vi "VCI_UsbDeviceReset.vi"(8 "error in (no error)":errorcluster caption="错误输入（无错误）", 9 "Reserved":u32, 10 "DevIndex":u32, 11 "DevType":T1=2 items=["USB-CAN"=2, "USB-CAN2"=3]) -> (0 "error out":errorcluster caption="错误输出", 3 "Return Val":T2=1 items=["OK"=1, "ERROR1"=0, "ERROR2"=-1])   [LabVIEW 2018, in "ControlCan.lvlib"]
uses:
  ControlCan.lvlib
  Return Val.ctl
  DevType.ctl
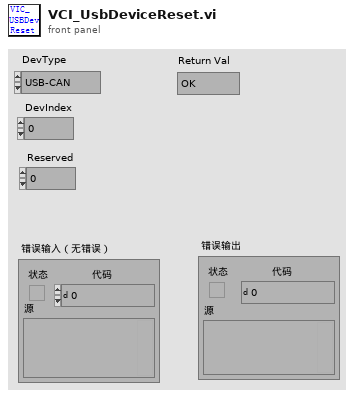
[diagram p1: front panel]
types:
  T1 = typedef "ControlCAN.lvlib/DevType.ctl" = u32
  T2 = typedef "ControlCAN.lvlib/Return Val.ctl" = i32
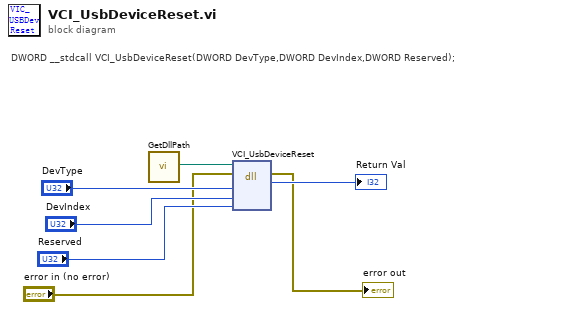
[diagram p0: block diagram]
diagram:
  # "DWORD __stdcall VCI_UsbDeviceReset(DWORD DevType,DWORD DevIndex,DWORD Reserved);"
  n1 = call "GetDllPath.vi"() -> ("DllPath"=w1:path)  [unwired: 1 in]
  n2 = dll-call lib="?" fn="VCI_UsbDeviceReset"(path in=w1, error in="error in (no error)", "DevType"="DevType", "DevIndex"="DevIndex", "Reserved"="Reserved") -> (error out=→"error out":errorcluster, "ReturnVal"=→"Return Val":i32)  [unwired: 4 in, 1 out]
